vi "transmitRFID v6 cw_query_rn16.vi"() -> ()   [LabVIEW 2015]
uses:
  <instrlib>/niUSRP/niUSRP Write Tx Data (CDB).vi
  Global_bits.vi
panel:
  out "ACK":bool
  out "bits":i16[](graph)
  out "RN16 array":i32[](array[numeric])
  in  "query":bool
  out "RFID Pushed":bool
  out "error out":errorcluster
  in  "Parameters Query":T1 {"Session" items=["S0", "S1", "S2", "S3"]; "Sel" items=["All", "All2", "~SL", "SL"]; "M" items=["M=1", "M=2", "M=4", "M=8"]}
  out "Wave Mag":dbl[](graph)
  out "Loop":i32
  in  "Symbol Rate [Hz]":dbl=500000.0 format="%#_13p"
  in  "Parameters Select":T2={"Target"=7, "Action"=0, "MemBank"=1, "truncate"=FALSE} {"MemBank" items=["00 RFU", "01 EPC", "10 TID", "11 User"]; "Action" items=["000", "001", "010", "011", "100", "101", "110", "111"]; "Target" items=["000 Inventoried (S0)", "001 Inventoried (S1)", "010 Inventoried (S2)", "011 Inventoried (S3)", "100 SL", "101 RFU", "110 RFU", "111 RFU"]}
  in  "Parameters Symbols":T3={"Tari"=8e-06, "PW"=0.5, "factor for \"1\" symbol"=0.5, "RTcal"=2.5, "TRcal"=3.0, "Delimiter"=1.4e-05} {"TRcal" min=1.1 max=3.0 step=0.1; "RTcal" min=2.5 max=3.0 step=0.1; "factor for \"1\" symbol" min=0.5 max=1.0 step=0.1; "PW" min=0.265 max=0.525 step=0.001; "Tari" format="%#_3p"}
  out "coerced IQ rate":dbl=100000.0 format="%#_6p"
  out "carrier frequency":dbl=100000.0 format="%#_6p"
  out "coerced gain":dbl format="%#_6f"
  in  "stop":bool
  in  "IQ rate":dbl=2000000.0 format="%#_6p"
  in  "carrier frequency":dbl=920000000.0 format="%#_6p"
  in  "gain":dbl format="%#_6f"
  in  "tx device names":refnum<k15>="192.168.20.13"
  # "Transmit RFID"
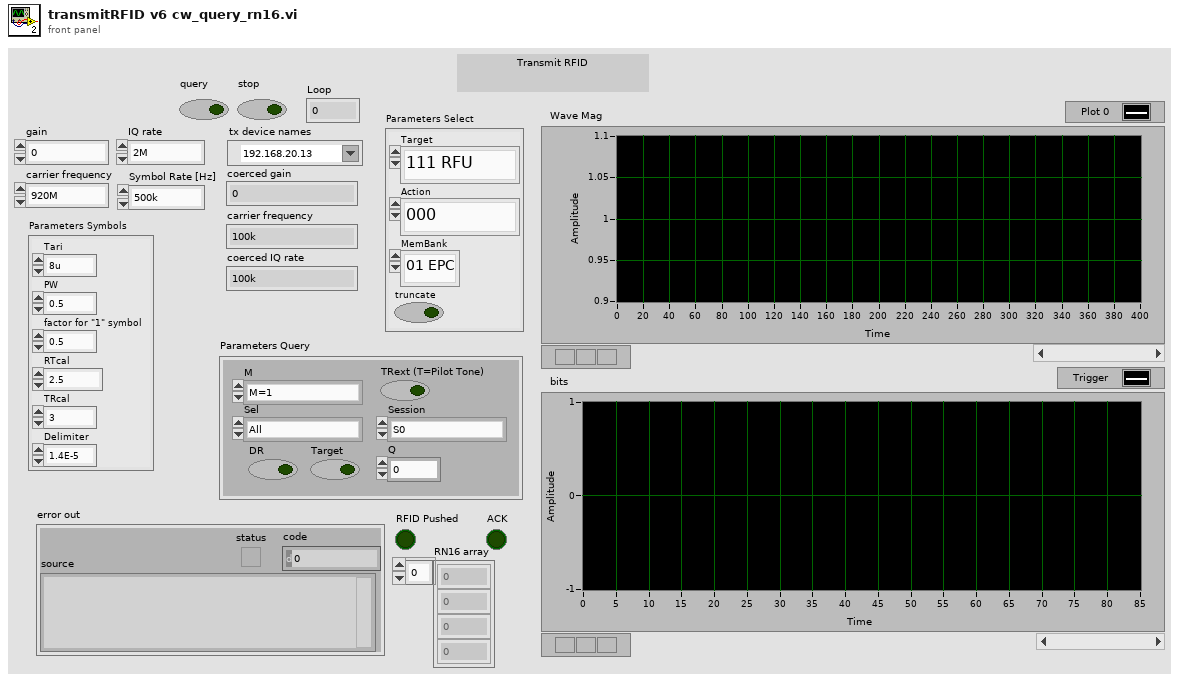
[diagram p1: front panel]
types:
  T1 = cluster{"DR":bool, "M":u16, "TRext (T=Pilot Tone)":bool, "Sel":u16, "Session":u16, "Q":u8, "Target":bool}
  T2 = cluster{"Target":u16, "Action":u16, "MemBank":u16, "truncate":bool}
  T3 = cluster{"Tari":dbl, "PW":dbl, "factor for \"1\" symbol":dbl, "RTcal":dbl, "TRcal":dbl, "Delimiter":dbl}
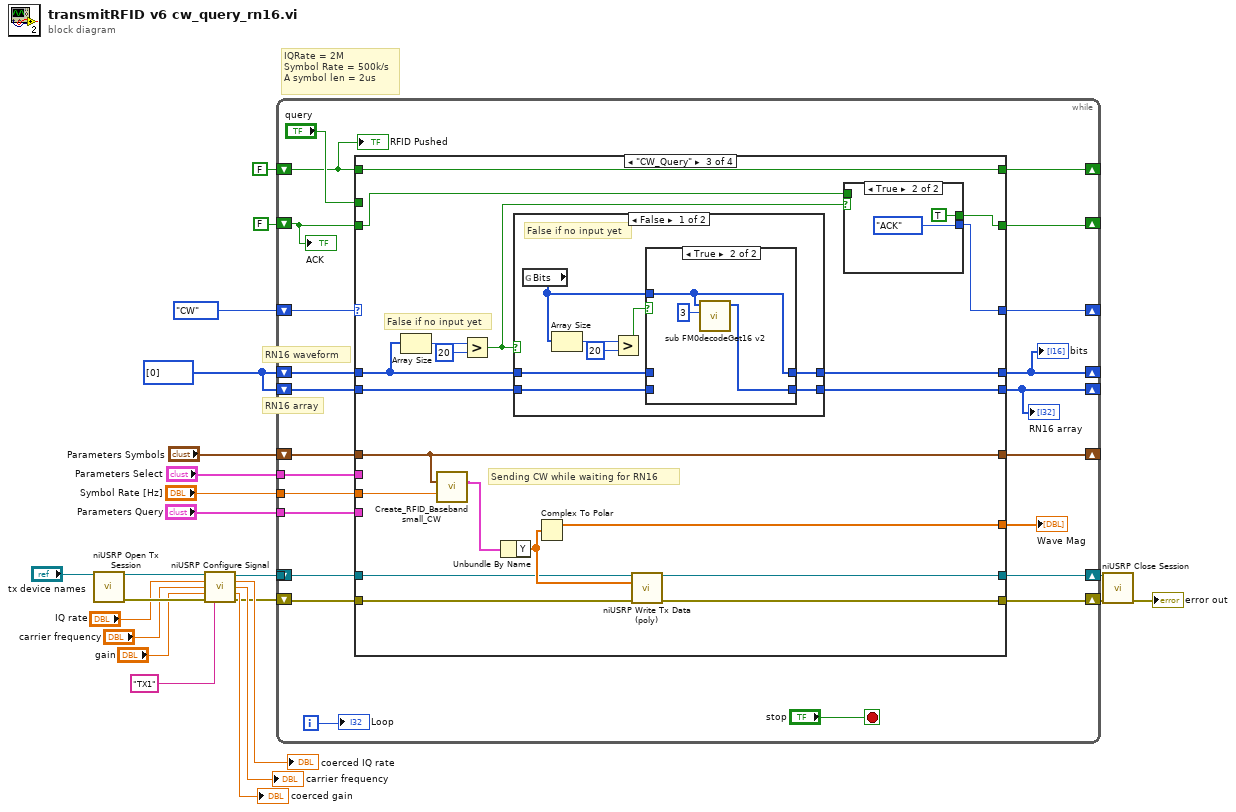
[diagram p0: block diagram]
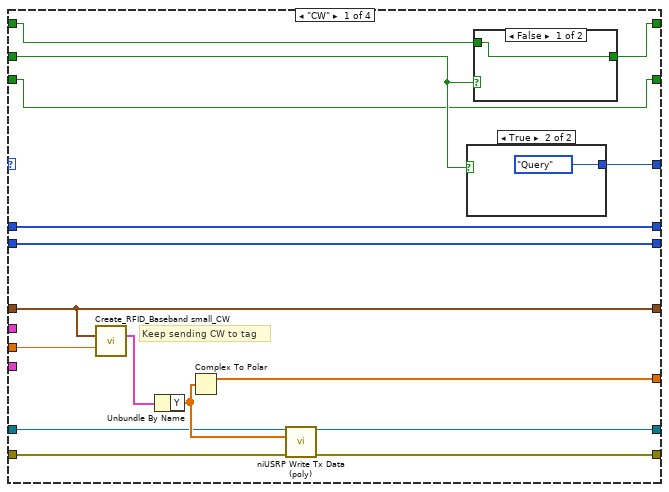
[diagram p2: hidden frame]
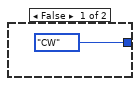
[diagram p4: hidden frame]
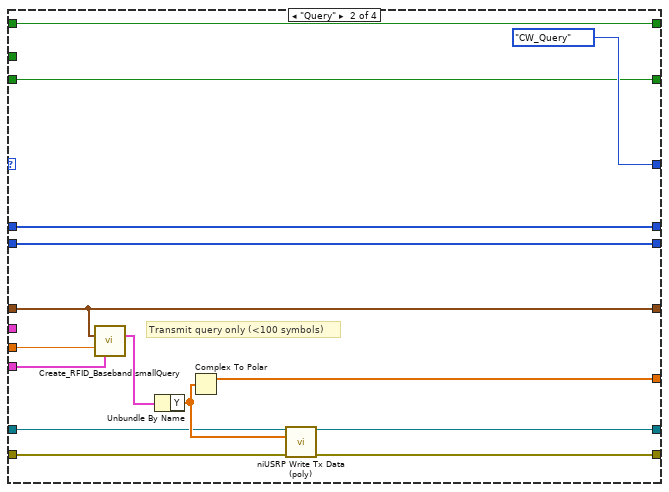
[diagram p5: hidden frame]
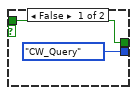
[diagram p6: hidden frame]
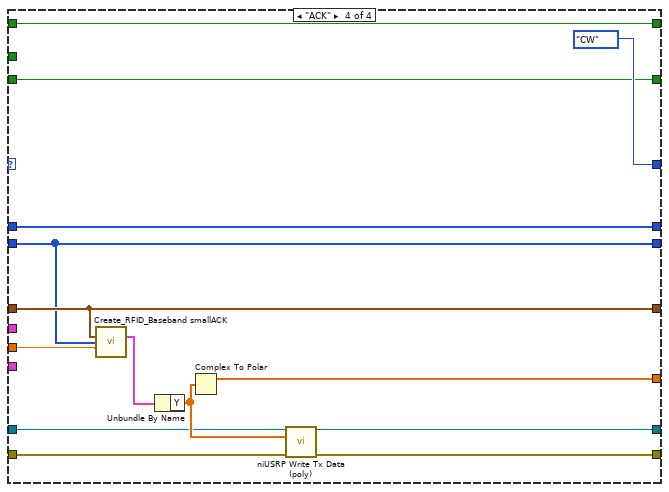
[diagram p9: hidden frame]
diagram:
  w3 = i16[] [0]
  # "IQRate = 2M\nSymbol Rate = 500k/s\nA symbol len = 2us"
  # "RN16 array"
  # "RN16 waveform"
  n1 = call <instrlib>:"niUSRP Open Tx Session.vi"("device names"="tx device names") -> ("session handle out"=w4:refnum<k15>, "error out"=w23:errorcluster)  [unwired: 13 in]
  n2 = call <instrlib>:"niUSRP Configure Signal.vi"("session handle"=w4, "IQ rate"="IQ rate", "carrier frequency"="carrier frequency", "gain"="gain", "error in (no error)"=w23, "active antenna"="TX1") -> ("session handle out"=w10:refnum<k15>, "coerced IQ rate"=→"coerced IQ rate":dbl, "coerced carrier frequency"=→"carrier frequency":dbl, "coerced gain"=→"coerced gain":dbl, "error out"=w9:errorcluster)  [unwired: 5 in]
  n3 = while {
    tunnel: "Parameters Select" -> [w39]
    tunnel: "Parameters Query" -> [w37]
    tunnel: w10 -> [w44]
    shift-right: [w42] -> w8
    shift-left: w9 -> [w43]
    shift-right: [w41] -> w6
    shift-left: _ -> [_]
    shift-right: [w34] -> _
    shift-left: enum16{"CW", "Query", "CW_Query", "ACK"}."CW" -> [w45]
    shift-right: [w36] -> _
    shift-left: "Parameters Symbols" -> [w40]
    tunnel: "Symbol Rate [Hz]" -> [w38]
    shift-right: [w32] -> _
    shift-left: w3 -> [w33]
    shift-right: [w31] -> _
    shift-left: w3 -> [w30]
    shift-right: [w27] -> _
    shift-left: FALSE ("query") -> [w26]
    shift-right: [w24] -> _
    shift-left: FALSE ("query") -> [w25]
    i -> [w46]
    stop <- "stop" stop-if-true
    n4 = case shown="\"CW_Query\"" w45 {
      tunnel: w44 -> [w61 w80 w100 w133]
      tunnel: w43 -> [w60 w79 w99 w132]
      tunnel: [w59 w78 w98 w131] -> w42
      tunnel: [w58 w77 w97 w130] -> w41
      tunnel: w40 -> [w56 w72 w88 w128]
      tunnel: w39 -> [_ _ _ _]
      tunnel: w38 -> [w55 w73 w87 w127]
      tunnel: w37 -> [_ w74 _ _]
      tunnel: [w56 w72 w88 w128] -> w36
      tunnel: [w57 w76 w96 w129] -> w29
      tunnel: [w53 enum16{"CW", "Query", "CW_Query", "ACK"}."CW_Query" w85 enum16{"CW", "Query", "CW_Query", "ACK"}."CW"] -> w34
      tunnel: "query" -> [w50 _ _ _]
      tunnel: w33 -> [w52 w71 w93 w124]
      tunnel: [w52 w71 w91 w124] -> w32
      tunnel: [w51 w70 w92 w125] -> w31
      tunnel: w30 -> [w51 w70 w90 w125]
      tunnel: [w49 w68 w84 w122] -> w27
      tunnel: w26 -> [w48 w68 w84 w122]
      tunnel: w25 -> [w47 w67 w83 w121]
      tunnel: [w47 w67 w82 w121] -> w24
      frame "CW" {
        # "Keep sending CW to tag"
        n5 = call "Create_RFID_Baseband small_CW.vi"("Parameters Symbols"=w56, "Symbol Rate [Hz]"=w55) -> ("complex waveform"=w54:cluster{"t0":dbl, "dt":dbl, "Y":cdb[]})  [unwired: 12 in, 1 out]
        n6 = Unbundle By Name(w54) -> ("Y"=w62:cdb[])
        n7 = Complex To Polar(r * e^(i*theta)=w62) -> (r=w57:dbl[])  [unwired: 1 out]
        n8 = call-poly <instrlib>:"niUSRP Write Tx Data (poly).vi"("session handle"=w61, "data"=w62, "error in (no error)"=w60) -> ("session handle out"=w58:refnum<k15>, "error out"=w59:errorcluster)  [unwired: 11 in]
        n9 = case shown="True" w50 {
          tunnel: [enum16{"CW", "Query", "CW_Query", "ACK"}."CW" enum16{"CW", "Query", "CW_Query", "ACK"}."Query"] -> w53
          frame False {
          }
          frame True {
          }
        }
        n10 = case shown="False" w50 {
          selector: w50 -> [_ w64]
          tunnel: [w63 w64] -> w49
          tunnel: w48 -> [w63 _]
          frame False {
          }
          frame True {
          }
        }
      }
      frame "Query" {
        # "Transmit query only (<100 symbols)"
        n11 = call "Create_RFID_Baseband smallQuery.vi"("Parameters Symbols"=w72, "Symbol Rate [Hz]"=w73, "Parameters Query"=w74) -> ("complex waveform"=w75:cluster{"t0":dbl, "dt":dbl, "Y":cdb[]})  [unwired: 11 in, 1 out]
        n12 = Unbundle By Name(w75) -> ("Y"=w81:cdb[])
        n13 = Complex To Polar(r * e^(i*theta)=w81) -> (r=w76:dbl[])  [unwired: 1 out]
        n14 = call-poly <instrlib>:"niUSRP Write Tx Data (poly).vi"("session handle"=w80, "data"=w81, "error in (no error)"=w79) -> ("session handle out"=w77:refnum<k15>, "error out"=w78:errorcluster)  [unwired: 11 in]
      }
      frame "CW_Query" {
        # "False if no input yet"
        # "Sending CW while waiting for RN16"
        n15 = Array Size(array=w93) -> (size(s)=w94:i32)
        n16 = call "Create_RFID_Baseband small_CW.vi"("Parameters Symbols"=w88, "Symbol Rate [Hz]"=w87) -> ("complex waveform"=w89:cluster{"t0":dbl, "dt":dbl, "Y":cdb[]})  [unwired: 12 in, 1 out]
        n17 = Greater?(x=w94, y=20) -> (0:w86:bool)
        n18 = Unbundle By Name(w89) -> ("Y"=w101:cdb[])
        n19 = case shown="False" w86 {
          tunnel: [w109 w120] -> w91
          tunnel: w93 -> [w110 w120]
          tunnel: [w107 w119] -> w92
          tunnel: w90 -> [w106 w119]
          frame False {
            # "False if no input yet"
            n20 = global read "Global_bits.vi" "Bits"() -> (w108:i16[])
            n21 = Array Size(array=w108) -> (size(s)=w113:i32)
            n22 = Greater?(x=w113, y=20) -> (0:w111:bool)
            n23 = case shown="True" w111 {
              tunnel: w110 -> [w115 _]
              tunnel: [w115 w117] -> w109
              tunnel: w108 -> [_ w117]
              tunnel: [w114 w118] -> w107
              tunnel: w106 -> [w114 _]
              frame False {
              }
              frame True {
                n24 = call "sub FM0decodeGet16 v2.vi"("threshold"=3, "RN16 waveform"=w117) -> ("RN16 array"=w118:i32[])  [unwired: 9 in]
              }
            }
          }
          frame True {
          }
        }
        n25 = Complex To Polar(r * e^(i*theta)=w101) -> (r=w96:dbl[])  [unwired: 1 out]
        n26 = call-poly <instrlib>:"niUSRP Write Tx Data (poly).vi"("session handle"=w100, "data"=w101, "error in (no error)"=w99) -> ("session handle out"=w97:refnum<k15>, "error out"=w98:errorcluster)  [unwired: 11 in]
        n27 = case shown="True" w86 {
          tunnel: [enum16{"CW", "Query", "CW_Query", "ACK"}."CW_Query" enum16{"CW", "Query", "CW_Query", "ACK"}."ACK"] -> w85
          tunnel: w83 -> [w102 _]
          tunnel: [w102 TRUE ("query")] -> w82
          frame False {
          }
          frame True {
          }
        }
      }
      frame "ACK" {
        n28 = call "Create_RFID_Baseband smallACK.vi"("Parameters Symbols"=w128, "RN16 array"=w125, "Symbol Rate [Hz]"=w127) -> ("complex waveform"=w126:cluster{"t0":dbl, "dt":dbl, "Y":cdb[]})  [unwired: 11 in, 1 out]
        n29 = Unbundle By Name(w126) -> ("Y"=w134:cdb[])
        n30 = Complex To Polar(r * e^(i*theta)=w134) -> (r=w129:dbl[])  [unwired: 1 out]
        n31 = call-poly <instrlib>:"niUSRP Write Tx Data (poly).vi"("session handle"=w133, "data"=w134, "error in (no error)"=w132) -> ("session handle out"=w130:refnum<k15>, "error out"=w131:errorcluster)  [unwired: 11 in]
      }
    }
    "RN16 array" <- w31
    "bits" <- w32
    "Wave Mag" <- w29
    "Loop" <- w46
    "RFID Pushed" <- w26
    "ACK" <- w25
  }
  n32 = call <instrlib>:"niUSRP Close Session.vi"("session handle"=w6, "error in (no error)"=w8) -> ("error out"=→"error out":errorcluster)  [unwired: 13 in]
